vi "Parse Algorithm Outputs.vi"(8 "error in (no error)":errorcluster, 11 "Algorithm Information":T1) -> (0 "error out":errorcluster, 4 "Q descriptions":string)   [LabVIEW 2013, in "QWTBLVLib.lvlib"]
doc: "Returns parsed informations about output quantities."
uses:
  QWTBLVLib.lvlib
  TD Algorithm Information.ctl
  TD Algorithm Information Input.ctl
  TD Algorithm Information Output.ctl
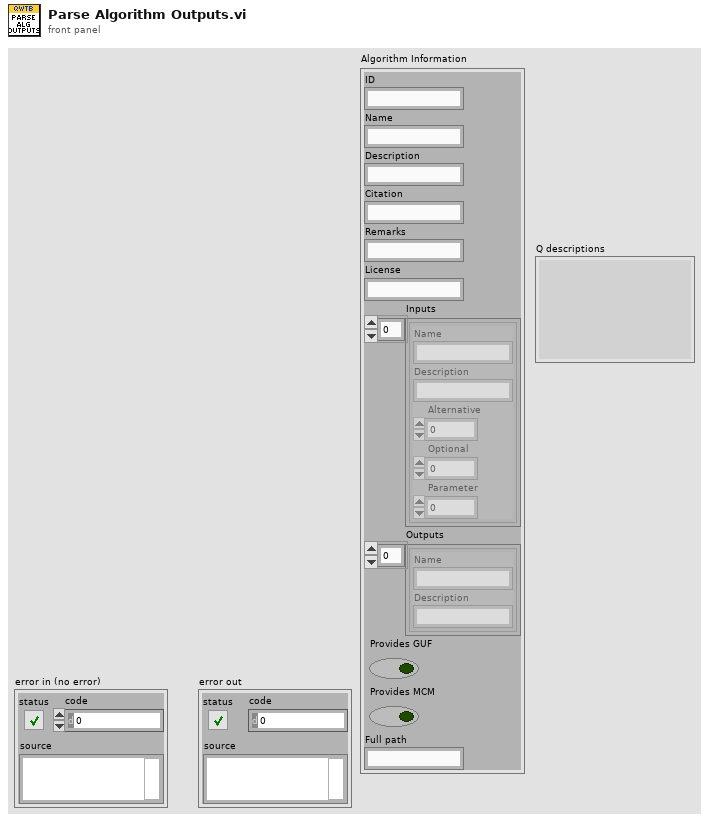
[diagram p1: front panel]
types:
  T1 = typedef "QWTBLVLib.lvlib/TD Algorithm Information.ctl" = cluster{"ID":string, "Name":string, "Description":string, "Citation":string, "Remarks":string, "License":string, "Inputs":T2[], "Outputs":T3[], "Provides GUF":bool, "Provides MCM":bool, "Full path":string}
  T2 = typedef "QWTBLVLib.lvlib/TD Algorithm Information Input.ctl" = cluster{"Name":string, "Description":string, "Alternative":i32, "Optional":i32, "Parameter":i32}
  T3 = typedef "QWTBLVLib.lvlib/TD Algorithm Information Output.ctl" = cluster{"Name":string, "Description":string}
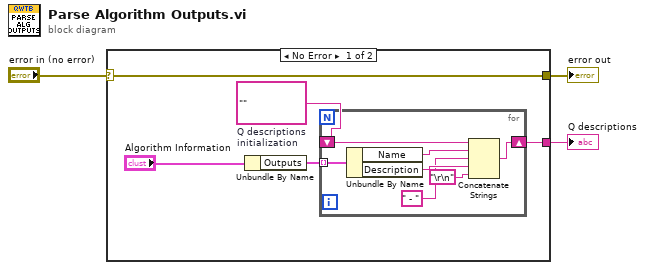
[diagram p0: block diagram]
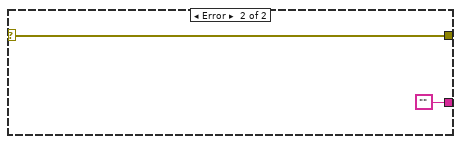
[diagram p2: hidden frame]
diagram:
  n1 = case shown="No Error" "error in (no error)" {
    selector: "error in (no error)" -> [w7 w17]
    tunnel: [w7 w17] -> w3
    tunnel: [w4 ""] -> w1
    frame No Error {
      w5 = ""  # Q descriptions initialization
      n2 = Unbundle By Name("Algorithm Information") -> ("Outputs"=w6:T3[])
      n3 = for {
        tunnel: w6 -> [w15] mode=indexing
        shift-right: [w11] -> w4
        shift-left: w5 -> [w10]
        n4 = Unbundle By Name(w15) -> ("Name"=w14:string, "Description"=w13:string)
        n5 = Concatenate Strings(w10, w14, " - " ("string"), w13, "\r\n") -> (w11:string)
      }
    }
    frame Error {
    }
  }
  "error out" <- w3
  "Q descriptions" <- w1
